vi "System@ProgramSection__Parameter.vi"(1 "ParamterIn":string) -> (0 "ParamterOut":string)   [LabVIEW 2020]
panel:
  in  "Name":string(combo)
  in  "Section":string(combo)
  in  "Confirm":bool
  # "System@ProgramSection $Section,$Section Name"
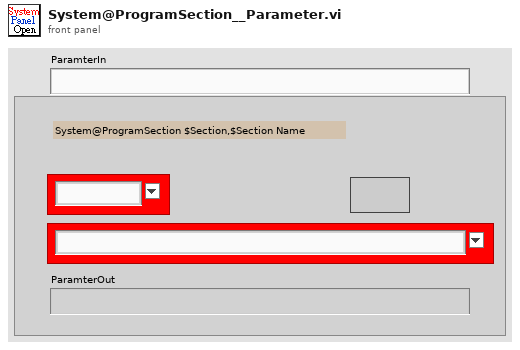
[diagram p1: front panel]
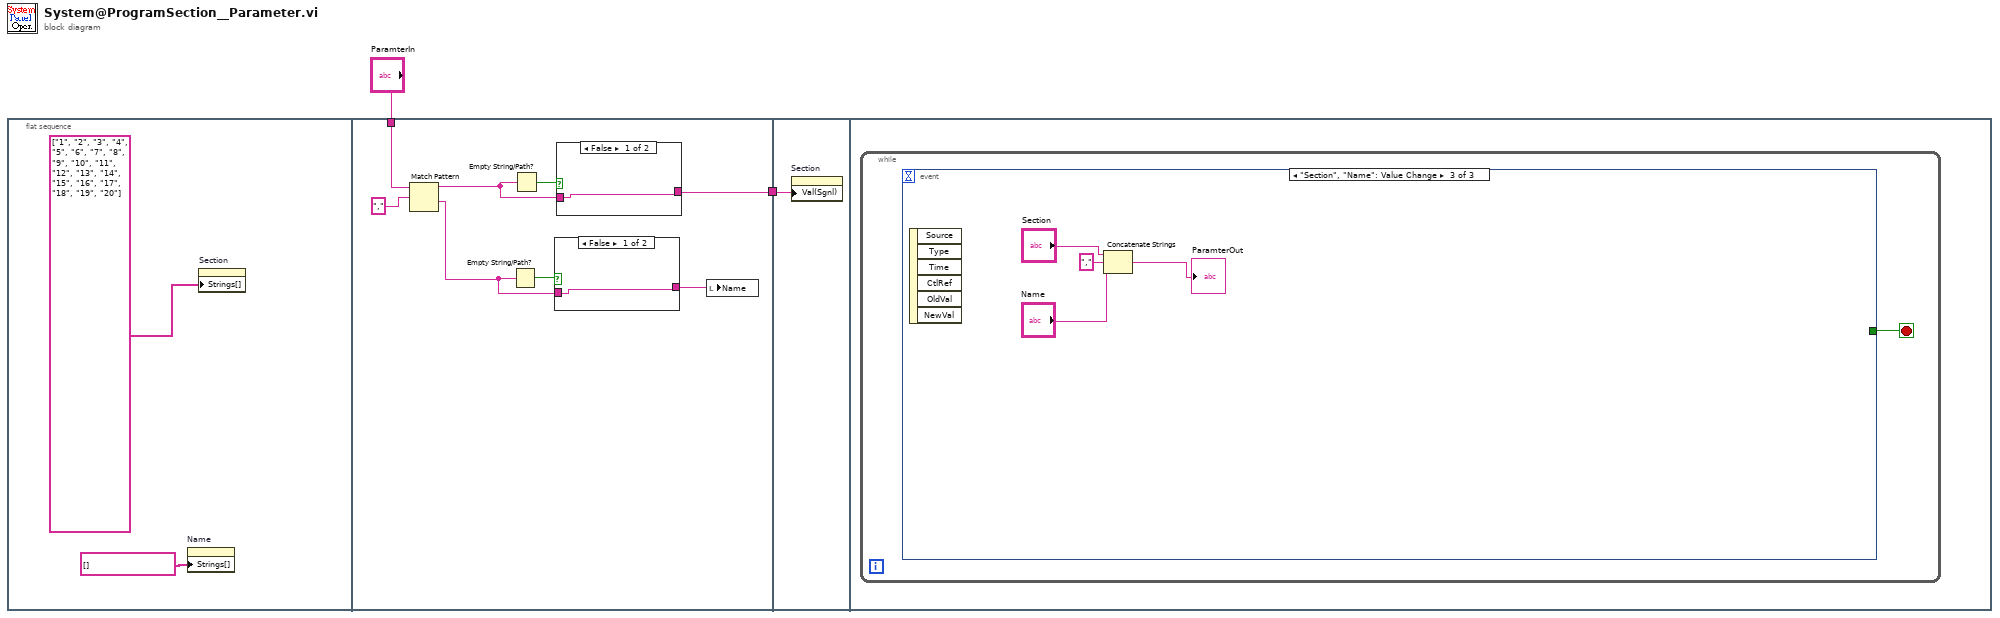
[diagram p0: block diagram]
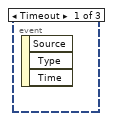
[diagram p4: hidden frame]
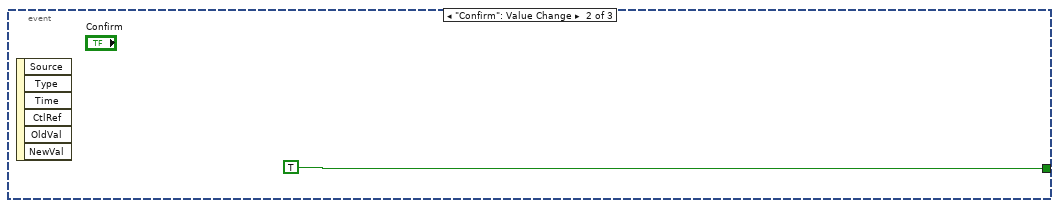
[diagram p5: hidden frame]
diagram:
  n1 = flat-sequence {
    tunnel: "ParamterIn" -> [w11]
    tunnel: [w6] -> w1
    tunnel: w1 -> [w17]
    frame #0 {
      n2 = property on="Name" class="CmbBox"("Strings[]"=string[] [] ("Strings []")) -> ()  [unwired: 2 in, 2 out]
      n3 = property on="Section" class="CmbBox"("Strings[]"=string[] ["1", "2", "3", "4", "5", "6", "7", "8", "9", "10", "11", "12", "13", "14", "15", "16", "17", "18", "19", "20"] ("Strings []")) -> ()  [unwired: 2 in, 2 out]
    }
    frame #1 {
      n4 = Match Pattern(string=w11, regular expression=",") -> (before substring=w9:string, after substring=w7:string)  [unwired: 1 in, 2 out]
      n5 = Empty String/Path?(string/path=w7) -> (empty?=w8:bool)
      n6 = Empty String/Path?(string/path=w9) -> (empty?=w12:bool)
      n7 = case shown="False" w8 {
        tunnel: w7 -> [w13 w14]
        tunnel: [w13 w14] -> w5
        frame False {
        }
        frame True {
        }
      }
      n8 = case shown="False" w12 {
        tunnel: w9 -> [w15 w16]
        tunnel: [w15 w16] -> w6
        frame False {
        }
        frame True {
        }
      }
      n9 = local write "Name"(w5) -> ()
    }
    frame #2 {
      n10 = property on="Section" class="CmbBox"("Val(Sgnl)"=w17) -> ()  [unwired: 2 in, 2 out]
    }
    frame #3 {
      n11 = while {
        stop <- w18 stop-if-true
        n12 = event shown="[2] \"Section\", \"Name\": Value Change" {
          selector: _ -> [_ _ _]
          dyn-events: _ -> [_ _ _]
          timeout: _ -> [_ _ _]
          tunnel: [_ TRUE _] -> w18
          event Timeout {
            n13 = event-data() -> ()  [unwired: 1 in, 3 out]
          }
          event "Confirm": Value Change {
            n14 = event-data() -> ()  [unwired: 1 in, 6 out]
          }
          event "Section", "Name": Value Change {
            n15 = event-data() -> ()  [unwired: 1 in, 6 out]
            n16 = Concatenate Strings("Section", "," ("string"), "Name") -> (→"ParamterOut":string)
          }
        }
      }
    }
  }
